vi "TimeStopTeste.vi"(11 "TimeInicio":u32) -> (3 "StopTeste":bool)   [LabVIEW 2019]
uses:
  TelaParametrosTeste/VariaveisParametros.vi
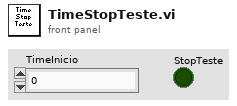
[diagram p1: front panel]
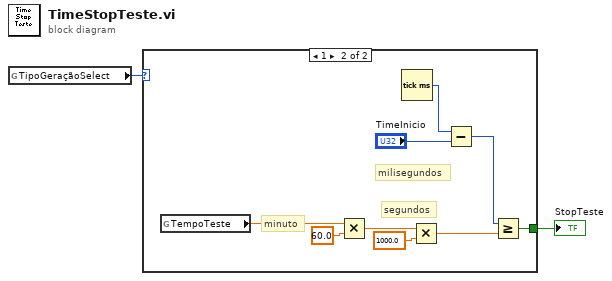
[diagram p0: block diagram]
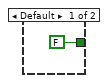
[diagram p2: hidden frame]
diagram:
  n1 = global read "VariaveisParametros.vi" "TipoGeraçãoSelect"() -> (w1:u16)
  n2 = case shown="1" w1 {
    tunnel: [FALSE w6] -> w2
    frame Default {
    }
    frame 1 {
      # "milisegundos"
      # "segundos"
      # "minuto"
      n3 = global read "VariaveisParametros.vi" "TempoTeste"() -> (w12:dbl)
      n4 = Multiply(x=w12, y=60.0) -> (x*y=w10:dbl)
      n5 = Tick Count (ms)() -> (millisecond timer value=w5:u32)
      n6 = Multiply(x=w10, y=1000.0) -> (x*y=w7:dbl)
      n7 = Subtract(x=w5, y="TimeInicio") -> (x-y=w8:u32)
      n8 = Greater Or Equal?(x=w8, y=w7) -> (x >= y?=w6:bool)
    }
  }
  "StopTeste" <- w2
